vi "P4CMDSub Extract Command Output.vi"(7 "bundled message":string) -> (6 "command output":string, 10 "command error":string)   [LabVIEW 2020, in "NI_SCC_P4CMD.lvlib"]
uses:
  <vilib>/SourceControl/Providers/P4CMD/NI_SCC_P4CMD.lvlib
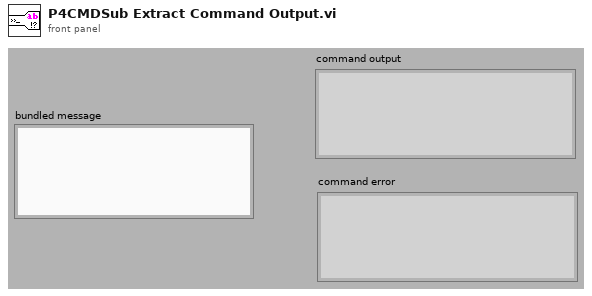
[diagram p1: front panel]
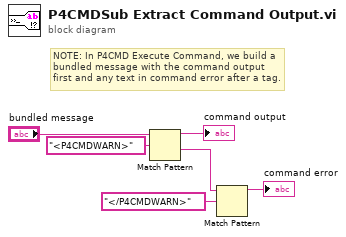
[diagram p0: block diagram]
diagram:
  # "NOTE: In P4CMD Execute Command, we build a bundled message with the command output first and any text in command error after a tag."
  n1 = Match Pattern(string="bundled message", regular expression="<P4CMDWARN>") -> (before substring=→"command output":string, after substring=w2:string)  [unwired: 1 in, 2 out]
  n2 = Match Pattern(string=w2, regular expression="</P4CMDWARN>") -> (before substring=→"command error":string)  [unwired: 1 in, 3 out]
